vi "_Subscr.Ver Test Module1.vi"() -> ()   [LabVIEW 2018, in "KATE_Lib.lvlib" / "Subscription.lvlib"]
uses:
  Subscription.lvlib
  Subscr.Subscription Request Info.ctl
  Queues/Q.Element.ctl
  Subscription.lvclass
  Queues/Queue Utils.lvlib
panel:
  in  "Disable":bool
  out "SubScrReq":T1[](array[typedef])
  in  "stop":bool
  in  "Bool":bool
  in  "Str":string
  in  "Host Q":string="Module 2"
  out "Bool  Subsc":bool
  out "Str Subsc":string
  in  "Subscribe to Bool":bool
  in  "Subscribe to Str":bool
  in  "Local Q":string="Module 1"
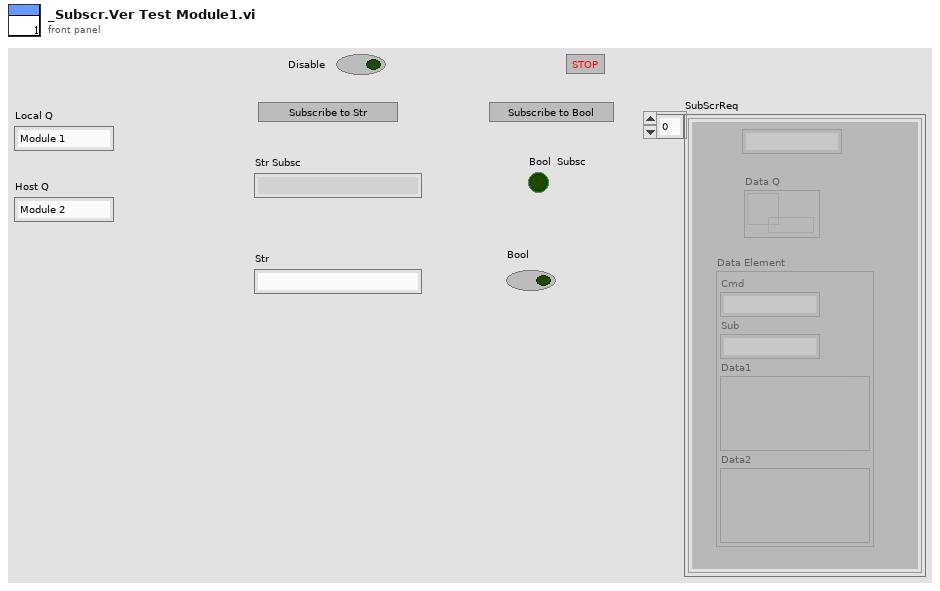
[diagram p1: front panel]
types:
  T1 = typedef "KATE_Lib.lvlib/Subscription.lvlib/Subscr.Subscription Request Info.ctl" = cluster{"Name":string, "Data Q":refnum<queue>, "Data Element":T2}
  T2 = typedef "KATE_Lib.lvlib/Queue Utils.lvlib/Q.Element.ctl" = cluster{"Cmd":string, "Sub":string, "Data1":variant, "Data2":variant}
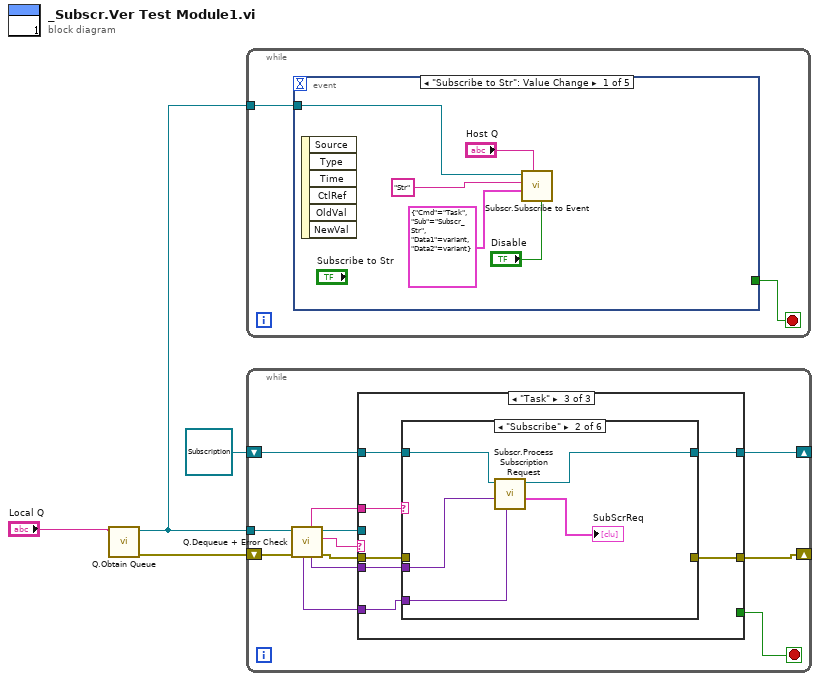
[diagram p0: block diagram]
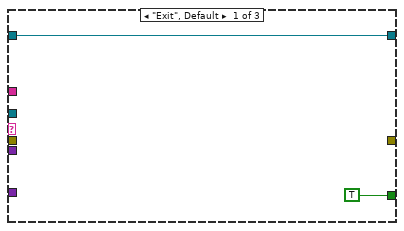
[diagram p2: hidden frame]
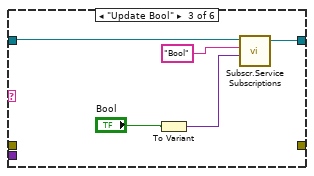
[diagram p5: hidden frame]
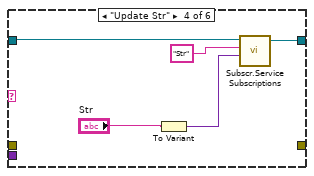
[diagram p6: hidden frame]
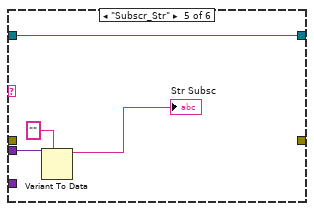
[diagram p7: hidden frame]
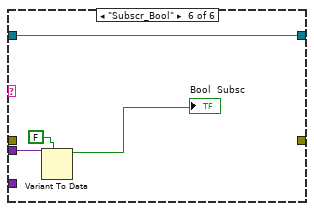
[diagram p8: hidden frame]
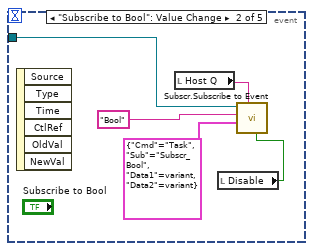
[diagram p9: hidden frame]
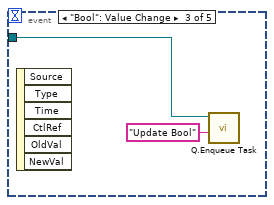
[diagram p10: hidden frame]
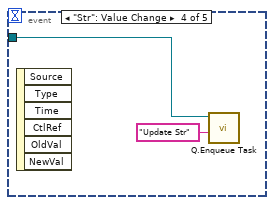
[diagram p11: hidden frame]
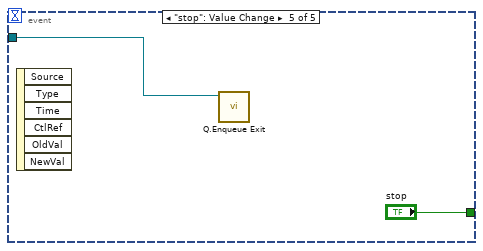
[diagram p12: hidden frame]
diagram:
  n1 = call "Q.Obtain Queue.vi"("Q Name"="Local Q") -> ("error out"=w1:errorcluster, "Q Out"=w3:refnum<queue>)  [unwired: 8 in, 1 out]
  n2 = while {
    tunnel: w3 -> [w6]
    stop <- w5 stop-if-true
    n3 = event shown="[0] \"Subscribe to Str\": Value Change" {
      selector: _ -> [_ _ _ _ _]
      dyn-events: _ -> [_ _ _ _ _]
      timeout: _ -> [_ _ _ _ _]
      tunnel: w6 -> [w11 w16 w18 w20 w21]
      tunnel: [_ _ _ _ "stop"] -> w5
      event "Subscribe to Str": Value Change {
        n4 = event-data() -> ()  [unwired: 1 in, 6 out]
        n5 = call "Subscr.Subscribe to Event.vi"("Disable"="Disable", "Source Q Name"="Host Q", "Data Element"=T2 {"Cmd"="Task", "Sub"="Subscr_Str", "Data1"=variant, "Data2"=variant}, "Event Name"="Str", "Local Q"=w11) -> ()  [unwired: 5 in, 2 out]
      }
      event "Subscribe to Bool": Value Change {
        n6 = event-data() -> ()  [unwired: 1 in, 6 out]
        n7 = local read "Host Q"() -> (w13:string)
        n8 = local read "Disable"() -> (w12:bool)
        n9 = call "Subscr.Subscribe to Event.vi"("Disable"=w12, "Source Q Name"=w13, "Data Element"=T2 {"Cmd"="Task", "Sub"="Subscr_Bool", "Data1"=variant, "Data2"=variant}, "Event Name"="Bool", "Local Q"=w16) -> ()  [unwired: 5 in, 2 out]
      }
      event "Bool": Value Change {
        n10 = event-data() -> ()  [unwired: 1 in, 6 out]
        n11 = call "Q.Enqueue Task.vi"("Task Name"="Update Bool", "Q In"=w18) -> ()  [unwired: 8 in, 2 out]
      }
      event "Str": Value Change {
        n12 = event-data() -> ()  [unwired: 1 in, 6 out]
        n13 = call "Q.Enqueue Task.vi"("Task Name"="Update Str", "Q In"=w20) -> ()  [unwired: 8 in, 2 out]
      }
      event "stop": Value Change {
        n14 = event-data() -> ()  [unwired: 1 in, 6 out]
        n15 = call "Q.Enqueue Exit.vi"("Q In"=w21) -> ()  [unwired: 9 in, 2 out]
      }
    }
  }
  n16 = while {
    tunnel: w3 -> [w34]
    shift-right: [w25] -> _
    shift-left: w1 -> [w26]
    shift-right: [w23] -> _
    shift-left: refnum<class "Subscription.lvclass"> refnum ("Subscription in") -> [w27]
    stop <- w28 stop-if-true
    n17 = call "Q.Dequeue + Error Check.vi"("Error In"=w26, "Q In"=w34) -> ("error out"=w24:errorcluster, "Cmd"=w32:string, "Q Out"=w33:refnum<queue>, "Data1"=w30:variant, "Sub"=w31:string, "Data2"=w29:variant)  [unwired: 4 in]
    n18 = case shown="\"Task\"" w32 {
      tunnel: w33 -> [_ _ _]
      tunnel: w31 -> [_ _ w44]
      tunnel: w30 -> [_ _ w43]
      tunnel: w29 -> [_ _ w38]
      tunnel: [TRUE _ _] -> w28
      tunnel: w27 -> [w35 w37 w42]
      tunnel: [_ _ w40] -> w25
      tunnel: w24 -> [_ _ w39]
      tunnel: [w35 w37 w41] -> w23
      frame "Exit", Default {
      }
      frame "Error" {
      }
      frame "Task" {
        n19 = case shown="\"Subscribe\"" w44 {
          tunnel: w43 -> [_ w48 _ _ w65 w69]
          tunnel: w42 -> [w46 w50 w55 w60 w62 w66]
          tunnel: [w46 w49 w56 w61 w62 w66] -> w41
          tunnel: [w45 _ _ _ _ _] -> w40
          tunnel: w39 -> [w45 _ _ _ _ _]
          tunnel: w38 -> [_ w47 _ _ _ _]
          frame Default {
          }
          frame "Subscribe" {
            n20 = call "Subscr.Process Subscription Request.vi"("Disable(Data2)"=w47, "Request Info (Data1)"=w48, "Subscription in"=w50) -> ("SubScrReq"=→"SubScrReq":T1[], "Subscription out"=w49:refnum<class "Subscription.lvclass">)  [unwired: 6 in, 1 out]
          }
          frame "Update Bool" {
            n21 = To Variant(anything="Bool") -> (Variant=w52:variant)
            n22 = call "Subscr.Service Subscriptions.vi"("Data"=w52, "Name"="Bool" ("Event Name"), "Subscription in"=w55) -> ("Subscription out"=w56:refnum<class "Subscription.lvclass">)  [unwired: 7 in, 1 out]
          }
          frame "Update Str" {
            n23 = To Variant(anything="Str") -> (Variant=w58:variant)
            n24 = call "Subscr.Service Subscriptions.vi"("Data"=w58, "Name"="Str" ("Event Name"), "Subscription in"=w60) -> ("Subscription out"=w61:refnum<class "Subscription.lvclass">)  [unwired: 7 in, 1 out]
          }
          frame "Subscr_Str" {
            n25 = Variant To Data(type="", Variant=w65) -> (data=→"Str Subsc":string)  [unwired: 1 in, 1 out]
          }
          frame "Subscr_Bool" {
            n26 = Variant To Data(type=FALSE ("Bool  Subsc"), Variant=w69) -> (data=→"Bool  Subsc":bool)  [unwired: 1 in, 1 out]
          }
        }
      }
    }
  }
